vi "Read Configuration.lvclass.vi"(8 "error in (no error)":errorcluster, 11 "Optical Spectrum Analyzer in":refnum<class "Optical Spectrum Analyzer.lvclass">) -> (0 "error out":errorcluster, 2 "Configuration.lvclass":refnum<class "Configuration.lvclass">, 3 "Optical Spectrum Analyzer out":refnum<class "Optical Spectrum Analyzer.lvclass">)   [LabVIEW 2018, in "Optical Spectrum Analyzer.lvlib" / "Optical Spectrum Analyzer.lvclass"]
uses:
  Optical Spectrum Analyzer.lvclass
  PPLs/Configuration/Configuration.lvlibp/Configuration.lvclass
  Optical Spectrum Analyzer.lvclass/Optical Spectrum Analyzer.ctl
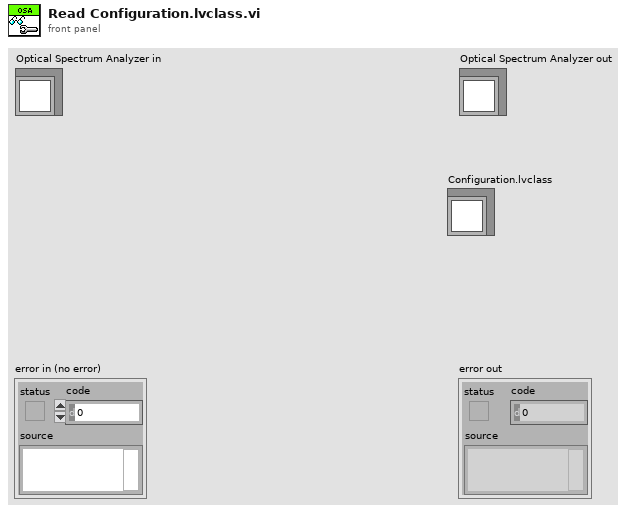
[diagram p1: front panel]
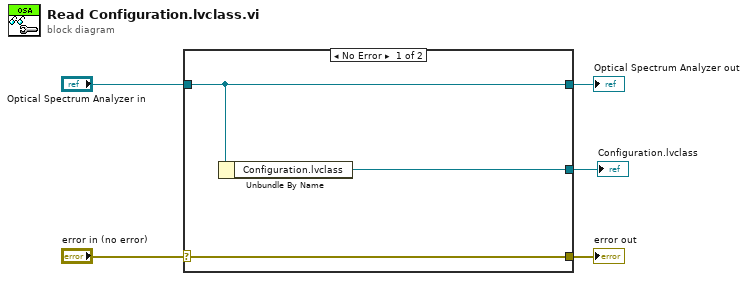
[diagram p0: block diagram]
diagram:
  n1 = case shown="No Error" "error in (no error)" {
    selector: "error in (no error)" -> [w8 w9]
    tunnel: [w8 w9] -> w4
    tunnel: [w7 w10] -> w2
    tunnel: "Optical Spectrum Analyzer in" -> [w7 w10]
    tunnel: [w6 _] -> w1
    frame No Error {
      n2 = Unbundle By Name(w7) -> ("Configuration.lvclass"=w6:refnum<class "Configuration.lvclass">)
    }
    frame Error {
    }
  }
  "error out" <- w4
  "Optical Spectrum Analyzer out" <- w2
  "Configuration.lvclass" <- w1
